vi "初始化.vi"(8 "error in (no error)":errorcluster caption="错误输入（无错误）", 11 "堆栈(DBL) 输入":refnum<class "堆栈(U64).lvclass"> caption="DNL_LabVIEW Object in") -> (0 "error out":errorcluster caption="错误输出", 3 "堆栈(DBL) 输出":refnum<class "堆栈(U64).lvclass"> caption="DNL_LabVIEW Object out")   [LabVIEW 2011, in "堆栈(U64).lvclass"]
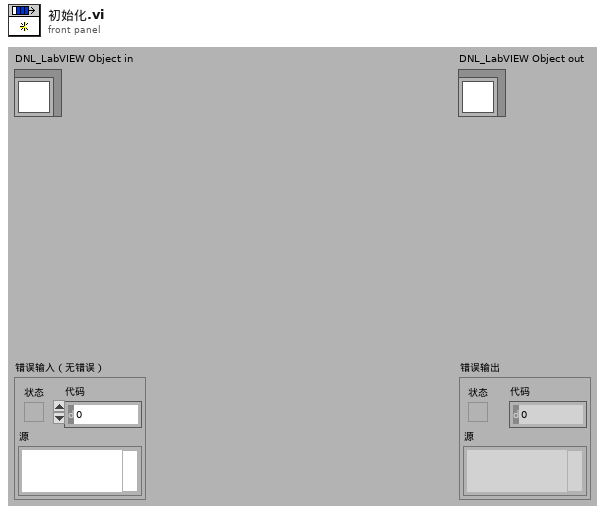
[diagram p1: front panel]
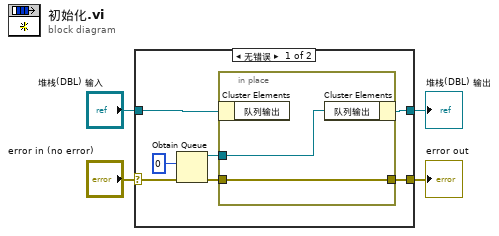
[diagram p0: block diagram]
diagram:
  n1 = case shown="无错误" "error in (no error)" {
    selector: "error in (no error)" -> [w7 w15]
    tunnel: [w5 w15] -> w3
    tunnel: [w8 w14] -> w1
    tunnel: "堆栈(DBL) 输入" -> [w10 w14]
    frame No Error {
      n2 = Obtain Queue(element data type=u64 0, error in (no error)=w7) -> (queue out=w9:refnum<queue>, error out=w6:errorcluster)  [unwired: 3 in, 1 out]
      n3 = in-place {
        in-place-border: w9 -> [w13]
        in-place-border: w6 -> [w12]
        in-place-border: [w12] -> w5
        n4 = in-place-cluster #1(w10) -> ()  [unwired: 1 out]
        n5 = in-place-cluster #1("队列输出"=w13) -> (w8:refnum<class "堆栈(U64).lvclass">)
      }
    }
    frame Error {
    }
  }
  "error out" <- w3
  "堆栈(DBL) 输出" <- w1
